vi "Create Evaluations.vi"(8 "error in (no error)":errorcluster, 11 "NF in":refnum<class "NF.lvclass">) -> (0 "error out":errorcluster, 1 "Evaluations Out":T1[](array[typedef]) {"Low Limit" format="%#_13g"; "SI Scaling" items=["femto"=-15, "pico"=-12, "nano"=-9, "micro"=-6, "milli"=-3, "percent"=-2, ""=0, "kilo"=3, "mega"=6, "giga"=9, "tera"=12]}, 3 "NF out":refnum<class "NF.lvclass">)   [LabVIEW 2018, in "NF.lvlib" / "NF.lvclass"]
uses:
  NF.lvclass
  C:/Sequence Automation/Plugins/Measurement Interface.lvlibp/Measurement Interface.lvclass
  Plugins/TestStand API Tools (TSAT).lvlibp/Evaluation Actions/Includes/Controls/TSAT Evaluation.ctl
  Plugins/TestStand API Tools (TSAT).lvlibp/Evaluation Actions/Includes/Controls/TSAT Eval SI Unit Scaling.ctl
  Plugins/TestStand API Tools (TSAT).lvlibp/Evaluation Actions/Includes/Controls/TSAT Evaluation Type.ctl
  Plugins/SeqAuto Evaluations.lvlibp/NF/NF Eval.lvclass
  Plugins/TestStand API Tools (TSAT).lvlibp/Evaluation Actions/TSAT Evaluation Actions.lvlib
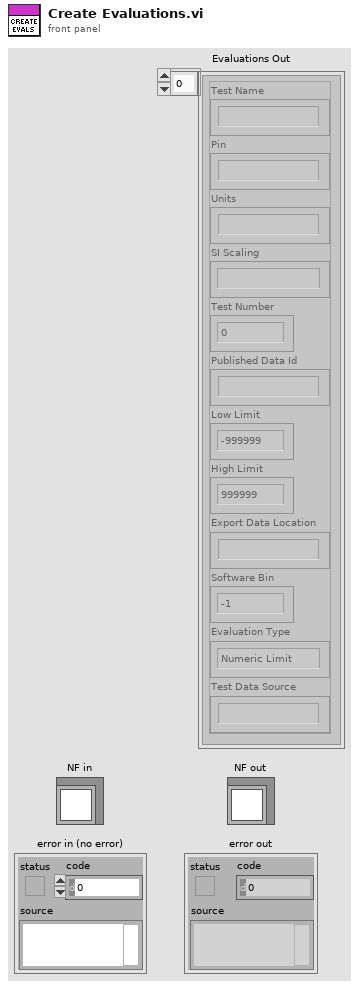
[diagram p1: front panel]
types:
  T1 = typedef "TestStand API Tools (TSAT).lvlibp/TSAT Evaluation Actions.lvlib/TSAT Evaluation.ctl" = cluster{"Test Name":string, "Pin":string, "Units":string, "SI Scaling":T2, "Test Number":i32, "Published Data Id":string, "Low Limit":dbl, "High Limit":dbl, "Export Data Location":string, "Software Bin":i64, "Evaluation Type":T3, "Test Data Source":string}
  T2 = typedef "TestStand API Tools (TSAT).lvlibp/TSAT Evaluation Actions.lvlib/TSAT Eval SI Unit Scaling.ctl" = i16
  T3 = typedef "TestStand API Tools (TSAT).lvlibp/TSAT Evaluation Actions.lvlib/TSAT Evaluation Type.ctl" = enum16{"Numeric Limit", "Pass/Fail", "None"}
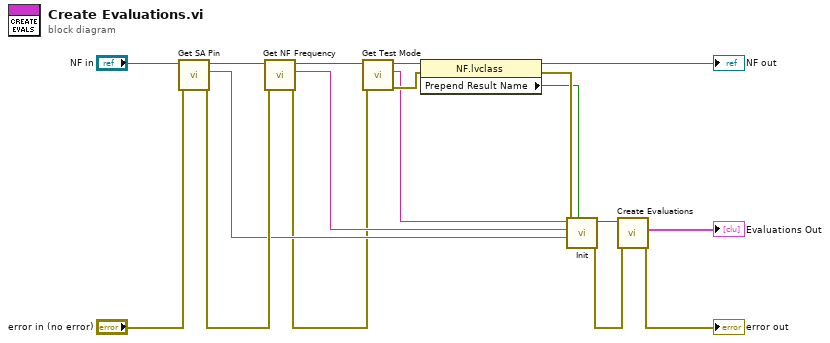
[diagram p0: block diagram]
diagram:
  n1 = call-dynamic "Get SA Pin.vi"("error in (no error)"="error in (no error)", "NF in"="NF in") -> ("error out"=w17:errorcluster, "SA Pin"=w14:string, "NF out"=w18:refnum<class "NF.lvclass">)  [unwired: 7 in]
  n2 = call-dynamic "Get NF Frequency.vi"("error in (no error)"=w17, "NF in"=w18) -> ("error out"=w13:errorcluster, "NF frequency"=w15:string, "NF out"=w7:refnum<class "NF.lvclass">)  [unwired: 7 in]
  n3 = call-dynamic "Get Test Mode.vi"("error in (no error)"=w13, "NF in"=w7) -> ("error out"=w8:errorcluster, "Test Mode"=w6:string, "NF out"=w3:refnum<class "NF.lvclass">)  [unwired: 7 in]
  n4 = property class="NF.lvclass"(reference=w3, error in=w8) -> (reference out=→"NF out":refnum<class "NF.lvclass">, error out=w4:errorcluster, "Prepend Result Name"=w1:bool)
  n5 = call "Init.vi"("Prepend Result Name"=w1, "error in (no error)"=w4, "SA Pin"=w14, "NF Freq (Hz)"=w15, "Measurement Name"=w6) -> ("error out"=w11:errorcluster, "NF out"=w12:refnum<class "NF Eval.lvclass">)  [unwired: 5 in]
  n6 = call-dynamic "Create Evaluations.vi"("error in (no error)"=w11, "IEvaluation in"=w12) -> ("error out"=→"error out":errorcluster, "Evaluations Out"=→"Evaluations Out":T1[])  [unwired: 7 in, 1 out]
